vi "Set ObjData.vi"(8 "error in (no error)":errorcluster, 10 "ObjData":T1={"Settings"={"Simulation"=FALSE, "Initial ErrReporting setting"=0, "Initial Measurement settings"={"Data Rate 9775"=3.0, "Data Rate 9215"=1200000.0, "Samples RMS 9215"=480000, "Samples RMS 9775"=3}, "Acquisition mode"=enum."3phase", "DemoMode"=FALSE, "RIO Device"=""}, "Public Events"={"DAQ_Engine.AsyncCmd Event"=refnum, "DAQ_Engine.AsyncMsg Event"=refnum, "stop process"=refnum, "DAQ_Engine.DAQStateChg Ev"=refnum, "DAQ_Engine.MeasSettingsChg Ev"=refnum, "DAQ_Engine.AcqModeChg Ev"=refnum}, "Dependency"={"Config"=refnum}, "ReadData-placeholder"={"Data"=0.0}, "VISA-placeholder"="", "MeasSettings"={"Data Rate 9775"=3.0, "Data Rate 9215"=1200000.0, "Samples RMS 9215"=480000, "Samples RMS 9775"=3}, "InverterDataAcqMode"=enum."3phase", "RawDaqDataQ"=refnum, "Private Events"={"PrivateAsync Ev"=refnum}, "DAQState Data"={"DAQState"=enum."Unknown", "vData"=variant}} {"Settings"."Initial ErrReporting setting" items=["DONTPRINT", "PRINTWARNINGS", "PRINTFATAL", "PRINTALL"]}, 11 "DAQ_Engine in":refnum<class "DAQ_Engine.lvclass">) -> (0 "error out":errorcluster, 3 "DAQ_Engine out":refnum<class "DAQ_Engine.lvclass">)   [LabVIEW 2019, in "DAQ_Engine.lvclass"]
doc: "Developed by Kevin Thompson\nkevin@thompsonengineering.net\n\nCopyright 2018\nThompson Engineering, LLC"
uses:
  DAQ_Engine.lvclass
  DataTypes/ObjData--cluster.ctl
  Config/Config.lvclass
  DataTypes/Settings--cluster.ctl
  Common/DataTypes/Measurement Config--cluster.ctl
  Common/DataTypes/Acquisition Mode--cluster.ctl
  DataTypes/Public Events--cluster.ctl
  Common/DataTypes/TD Async CmdMsg EventData--cluster.ctl
  DataTypes/DAQStateChg EvData--cluster.ctl
  DataTypes/DAQStateEvData--cluster.ctl
  Common/DataTypes/DAQState--enum.ctl
  DataTypes/DAQMeasSettingsChg EvData--cluster.ctl
  DataTypes/DAQMeasSettingsEvData--cluster.ctl
  DataTypes/DAQAcqModeChg EvData--cluster.ctl
  DataTypes/Dependency--cluster.ctl
  DataTypes/Read Data--cluster.ctl
  Common/DataTypes/RawDAQDataQRef--cluster.ctl
  Common/DataTypes/RawDAQData--cluster.ctl
  Common/DataTypes/RawChannelData--cluster.ctl
  DataTypes/Private Events--cluster.ctl
  DAQ_Engine.lvclass/DAQ_Engine.ctl
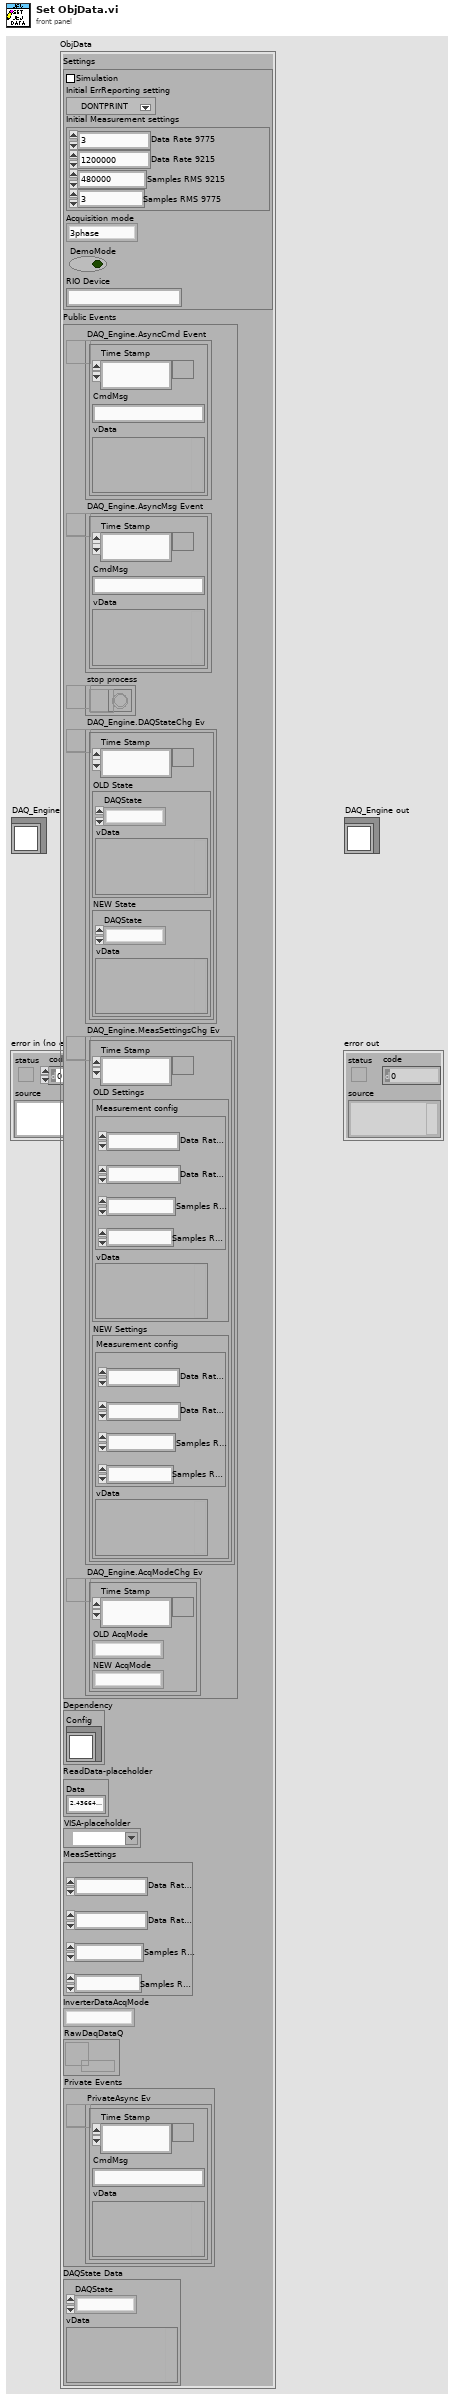
[diagram p1: front panel]
types:
  T1 = typedef "DAQ_Engine.lvclass/ObjData--cluster.ctl" = cluster{"Settings":T2, "Public Events":T5, "Dependency":T6, "ReadData-placeholder":T7, "VISA-placeholder":refnum<visa-resource-name>, "MeasSettings":T3, "InverterDataAcqMode":T4, "RawDaqDataQ":T8, "Private Events":T9, "DAQState Data":T10}
  T2 = typedef "DAQ_Engine.lvclass/Settings--cluster.ctl" = cluster{"Simulation":bool, "Initial ErrReporting setting":i32, "Initial Measurement settings":T3, "Acquisition mode":T4, "DemoMode":bool, "RIO Device":string}
  T3 = typedef "Measurement Config--cluster.ctl" = cluster{"Data Rate 9775":dbl, "Data Rate 9215":dbl, "Samples RMS 9215":u32, "Samples RMS 9775":u32}
  T4 = typedef "Acquisition Mode--cluster.ctl" = enum16{"3phase", "Single"}
  T5 = typedef "DAQ_Engine.lvclass/Public Events--cluster.ctl" = cluster{"DAQ_Engine.AsyncCmd Event":refnum<user-event>, "DAQ_Engine.AsyncMsg Event":refnum<user-event>, "stop process":refnum<user-event>, "DAQ_Engine.DAQStateChg Ev":refnum<user-event>, "DAQ_Engine.MeasSettingsChg Ev":refnum<user-event>, "DAQ_Engine.AcqModeChg Ev":refnum<user-event>}
  T6 = typedef "DAQ_Engine.lvclass/Dependency--cluster.ctl" = cluster{"Config":refnum<class "Config.lvclass">}
  T7 = typedef "DAQ_Engine.lvclass/Read Data--cluster.ctl" = cluster{"Data":dbl}
  T8 = typedef "RawDAQDataQRef--cluster.ctl" = refnum<queue>
  T9 = typedef "DAQ_Engine.lvclass/Private Events--cluster.ctl" = cluster{"PrivateAsync Ev":refnum<user-event>}
  T10 = typedef "DAQ_Engine.lvclass/DAQStateEvData--cluster.ctl" = cluster{"DAQState":T11, "vData":variant}
  T11 = typedef "DAQState--enum.ctl" = enum16{"Unknown", "Stopped", "Running", "Error"}
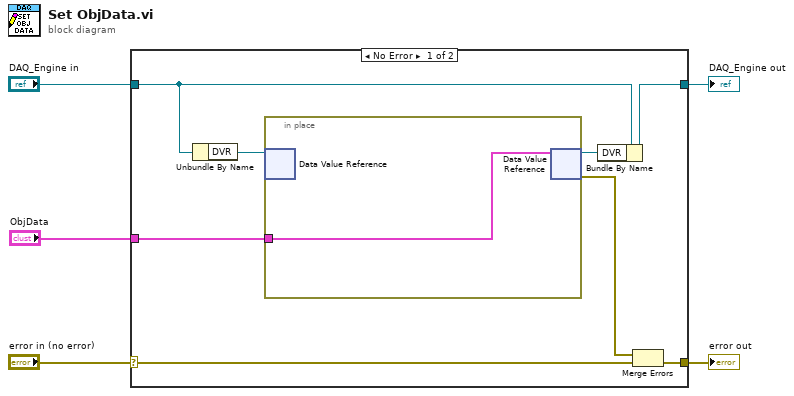
[diagram p0: block diagram]
diagram:
  n1 = case shown="No Error" "error in (no error)" {
    selector: "error in (no error)" -> [w13 w15]
    tunnel: [w7 w15] -> w4
    tunnel: [w9 w16] -> w2
    tunnel: "DAQ_Engine in" -> [w12 w16]
    tunnel: "ObjData" -> [w8 _]
    frame No Error {
      n2 = Unbundle By Name(w12) -> ("DVR"=w11:refnum<data-value>)
      n3 = in-place {
        in-place-border: w8 -> [w14]
        n4 = in-place-dvr #1(w11) -> ()  [unwired: 2 out]
        n5 = in-place-dvr #1(w14) -> (w10:refnum<data-value>, w6:errorcluster)
      }
      n6 = Bundle By Name(cluster=w12, "DVR"=w10) -> (w9:refnum<class "DAQ_Engine.lvclass">)
      n7 = Merge Errors(w6, w13) -> (w7:errorcluster)
    }
    frame Error {
    }
  }
  "error out" <- w4
  "DAQ_Engine out" <- w2
